vi "Get Channels Test.vi"() -> (0 "error out":errorcluster, 3 "channels match":bool)   [LabVIEW 2014, in "Modbus Tests.lvlib"]
uses:
  Modbus Tests.lvlib
  module/configuration/Modbus Module configuration.lvclass
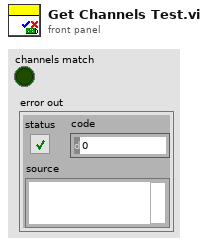
[diagram p1: front panel]
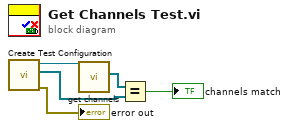
[diagram p0: block diagram]
diagram:
  n1 = call "Create Test Configuration.vi"() -> ("error out"=→"error out":errorcluster, "Channels"=w2:refnum<class "Modbus Module Channel.lvclass">[], "Module configuration"=w3:refnum<class "Modbus Module configuration.lvclass">)  [unwired: 9 in]
  n2 = call-dynamic "get channels.vi"("Modbus Slave configuration in"=w3) -> ("channels"=w5:refnum<class "TBM channel.lvclass">[])  [unwired: 9 in, 1 out]
  n3 = Equal?(x=w5, y=w2) -> (x = y?=→"channels match":bool)
